vi "START8FIXSTRING.vi"() -> ()   [LabVIEW 2024]
uses:
  <vilib>/Utility/file.llb/Read Delimited Spreadsheet (DBL).vi
panel:
  out "Boolean 2":bool
  in  "stop 2":bool
  in  "Flow Rate Upper Limit":dbl
  in  "Flow Rate Lower Limit":dbl
  in  "Initial RPM":dbl
  in  "Desired Flow Rate":dbl
  out "Waveform Chart 3":dbl[](graph)
  out "Waveform Chart 2":dbl[](graph)
  out "Flow Rate":dbl[](graph)
  in  "Color Box":u32(colorbox)
  # "Blood Flow Rate"
  # "Flow Rate (L/min)"
  # "Initial LVAD Speed (RPM)"
  # "Desired Flow Rate (L/min)"
  # "LVAD Speed"
  # "Upper Flow Rate Limit (L/min)"
  # "Lower Flow Rate Limit (L/min)"
  # "Speed (RPM)"
  # "Optimal Flow State"
  # "Right Heart ?????????"
  # "Displacement(????)"
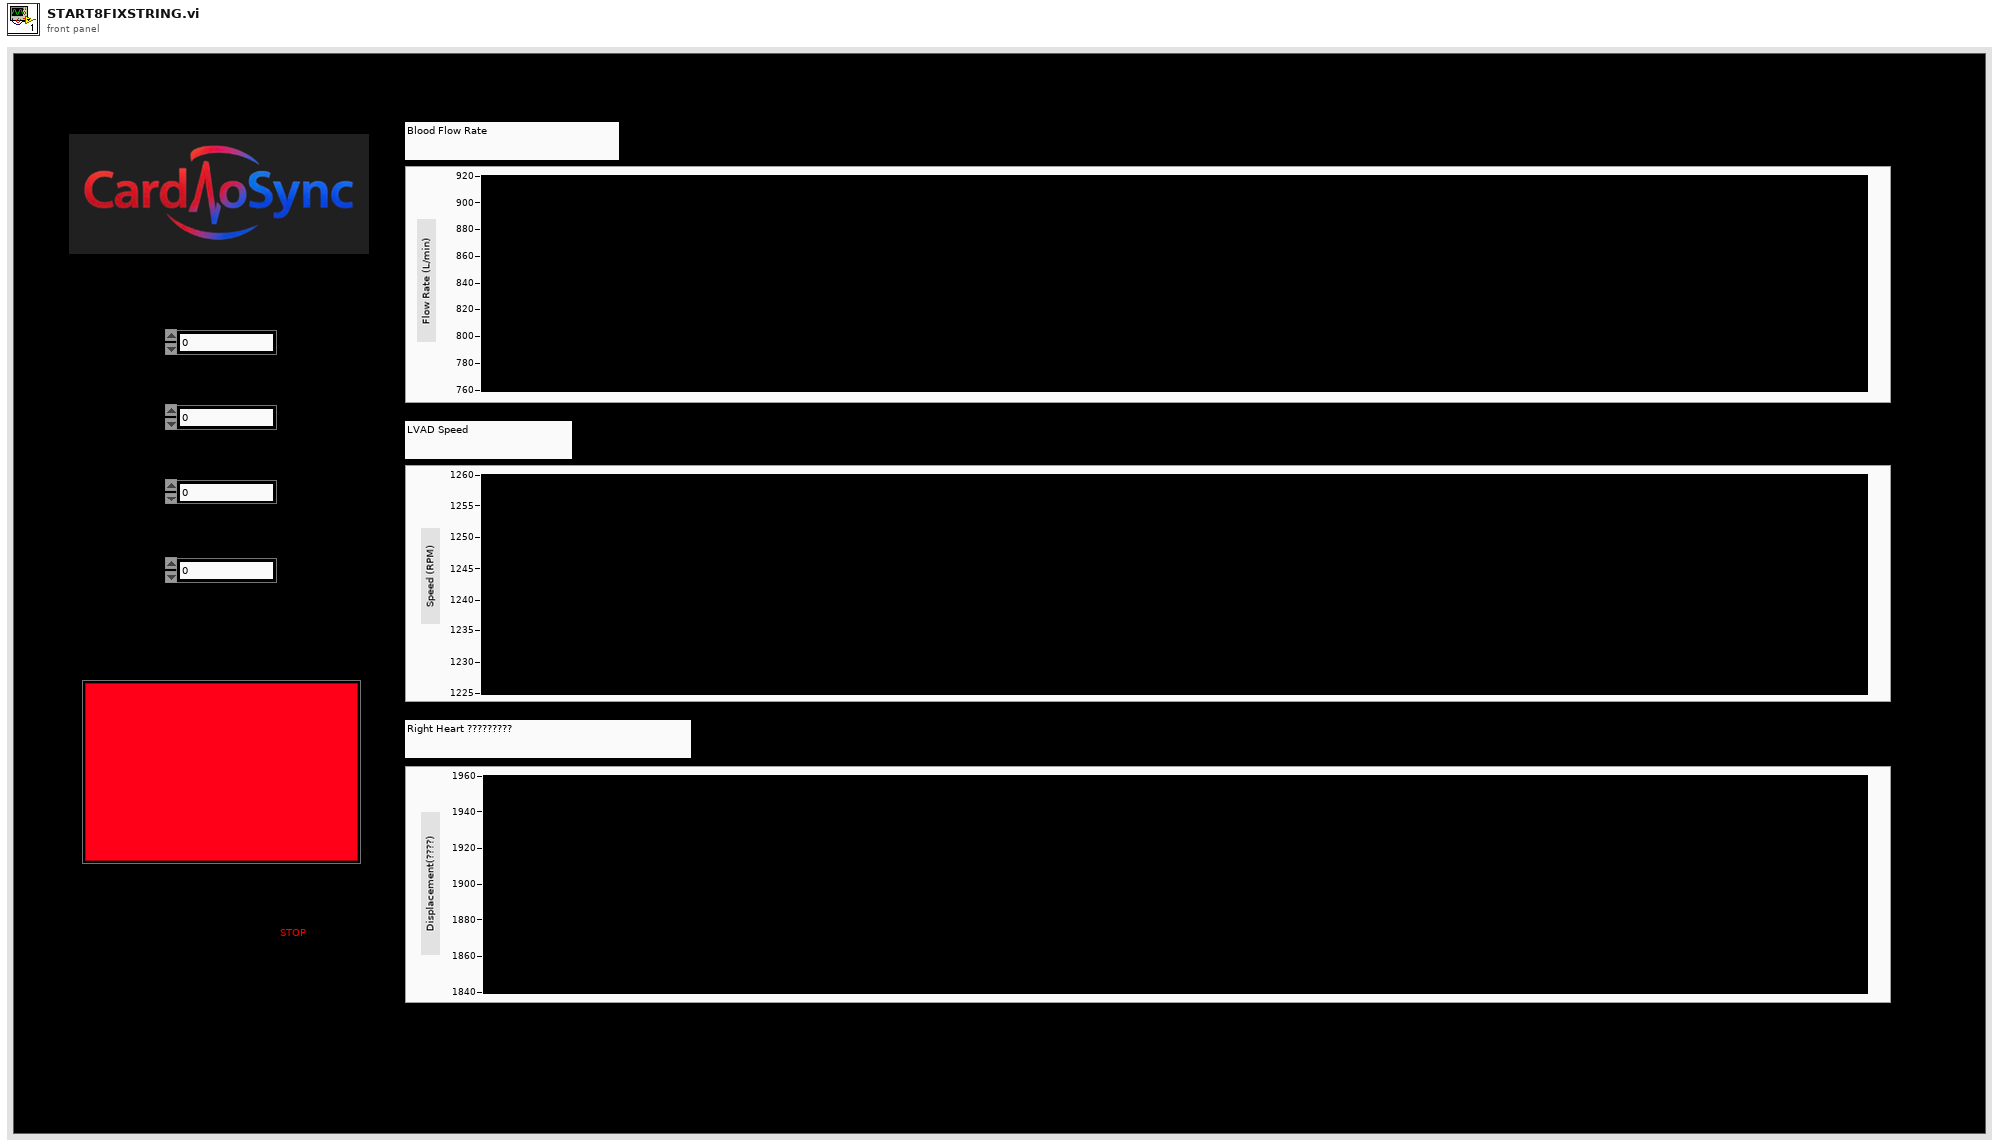
[diagram p1: front panel]
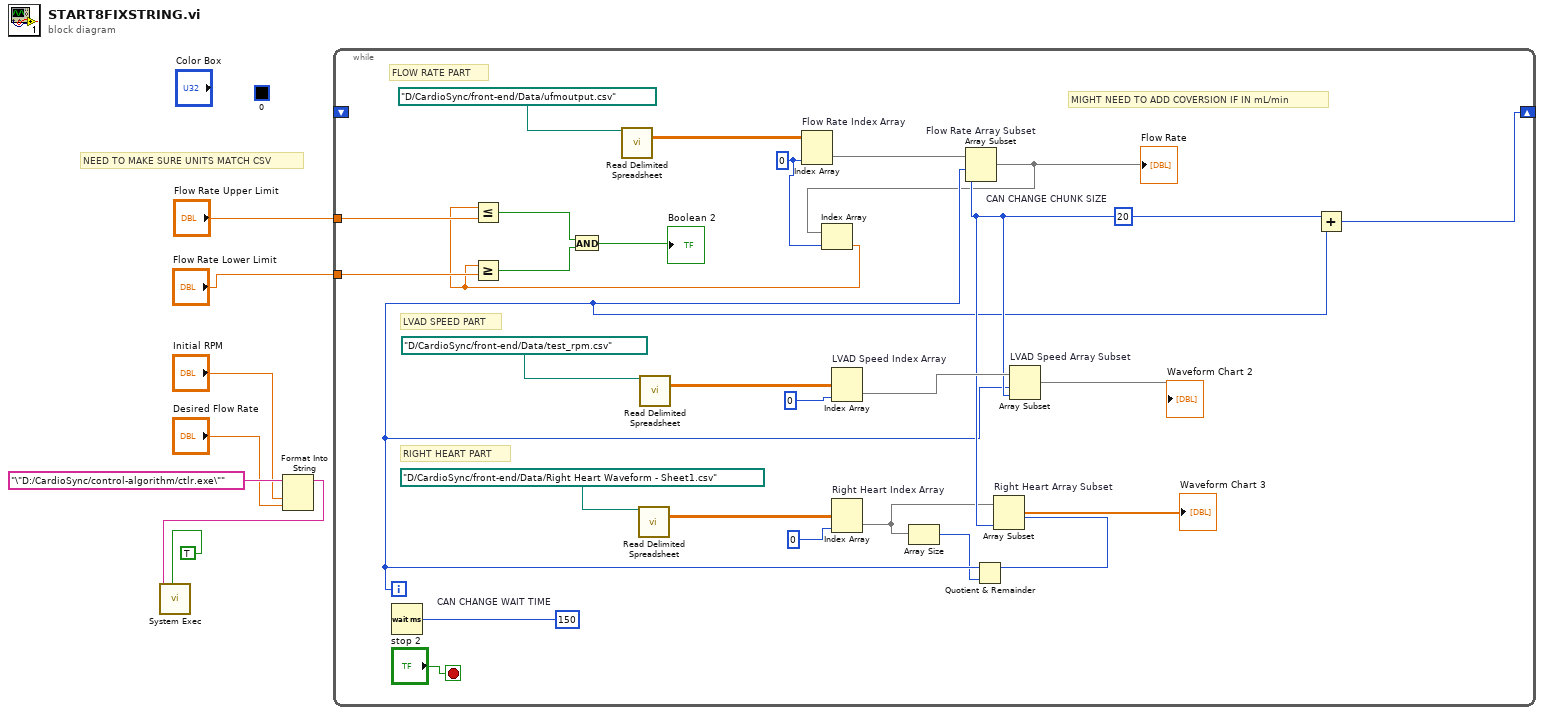
[diagram p0: block diagram]
diagram:
  (unwired) u32 0 ("Color Box 2")
  # "NEED TO MAKE SURE UNITS MATCH CSV"
  n1 = Format Into String(initial string="\"D:/CardioSync/control-algorithm/ctlr.exe\"", "Initial RPM", "Desired Flow Rate") -> (resulting string=w4:string)  [unwired: 2 in, 1 out]
  n2 = call <vilib>:"System Exec.vi"("wait until completion? (T)"=TRUE, "command line"=w4) -> ()  [unwired: 6 in, 4 out]
  n3 = while {
    shift-right: [w31] -> _
    shift-left: _ -> [_]
    tunnel: "Flow Rate Upper Limit" -> [w16]
    tunnel: "Flow Rate Lower Limit" -> [w15]
    i -> [w19]
    stop <- "stop 2" stop-if-true
    w32 = u32 150  # CAN CHANGE WAIT TIME
    w24 = 20  # CAN CHANGE CHUNK SIZE
    w11 = 0 ("disabled index (col)")
    # "MIGHT NEED TO ADD COVERSION IF IN mL/min"
    # "RIGHT HEART PART"
    # "LVAD SPEED PART"
    # "FLOW RATE PART"
    n4 = Wait (ms)(milliseconds to wait=w32) -> ()  [unwired: 1 out]
    n5 = call-poly <vilib>:"Read Delimited Spreadsheet.vi"("file path (dialog if empty)"=path "D:/CardioSync/front-end/Data/ufmoutput.csv") -> ("all rows"=w34:dbl[][])  [unwired: 9 in, 5 out]
    n6 = call-poly <vilib>:"Read Delimited Spreadsheet.vi"("file path (dialog if empty)"=path "D:/CardioSync/front-end/Data/Right Heart Waveform - Sheet1.csv") -> ("all rows"=w25:dbl[][])  [unwired: 9 in, 5 out]
    n7 = call-poly <vilib>:"Read Delimited Spreadsheet.vi"("file path (dialog if empty)"=path "D:/CardioSync/front-end/Data/test_rpm.csv") -> ("all rows"=w28:dbl[][])  [unwired: 9 in, 5 out]
    n8 = Index Array "Flow Rate Index Array"(array=w34, index (col)=w11) -> (element=w33:dbl[])  [unwired: 1 in]
    n9 = Index Array "LVAD Speed Index Array"(array=w28, index (col)=0 ("disabled index (col)")) -> (element=w27:dbl[])  [unwired: 1 in]
    n10 = Index Array "Right Heart Index Array"(array=w25, index (col)=0 ("disabled index (col)")) -> (element=w20:dbl[])  [unwired: 1 in]
    n11 = Array Size(array=w20) -> (size(s)=w18:i32)
    n12 = Array Subset "Flow Rate Array Subset"(array=w33, index=w19, length=w24) -> (w12:dbl[])
    "Flow Rate" <- w12
    n13 = Index Array(array=w12, index=w11) -> (element=w10:dbl)
    n14 = Less Or Equal?(x=w10, y=w16) -> (x <= y?=w14:bool)
    n15 = Greater Or Equal?(x=w10, y=w15) -> (x >= y?=w13:bool)
    n16 = And(x=w14, y=w13) -> (x .and. y?=→"Boolean 2":bool)
    n17 = Quotient & Remainder(x=w19, y=w18) -> (x-y*floor(x/y)=w17:i32)  [unwired: 1 out]
    n18 = Array Subset "Right Heart Array Subset"(array=w20, index=w17, length=w24) -> (→"Waveform Chart 3":dbl[])
    n19 = Array Subset "LVAD Speed Array Subset"(array=w27, index=w19, length=w24) -> (→"Waveform Chart 2":dbl[])
    n20 = Add(x=w24, y=w19) -> (x+y=w31:i32)
  }
